vi "DAC_C2_Continu.vi"() -> ()   [LabVIEW 2015]
uses:
  <vilib>/DAQmx/read.llb/DAQmx Read (Analog DBL 1Chan 1Samp).vi
  <vilib>/DAQmx/create/channels.llb/DAQmx Create Channel (AI-Voltage-Basic).vi
  <vilib>/DAQmx/configure/timing.llb/DAQmx Timing (Sample Clock).vi
  <vilib>/DAQmx/miscellaneous.llb/DAQmx Fill In Error Info.vi
panel:
  in  "stop":bool
  out "data":dbl(graph)
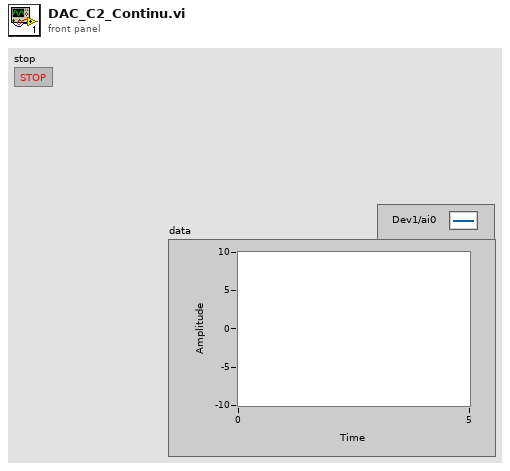
[diagram p1: front panel]
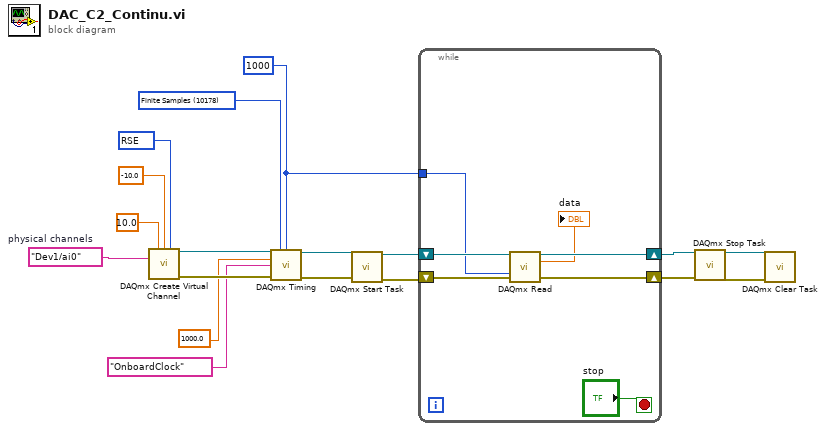
[diagram p0: block diagram]
diagram:
  w5 = 1000 ("samples per channel")
  w14 = 10178 items=["Finite Samples"=10178, "Continuous Samples"=10123, "Hardware Timed Single Point"=12522] ("sample mode")
  w15 = tag "Dev1/ai0"  # physical channels
  w18 = 10083 items=["Default"=-1, "RSE"=10083, "NRSE"=10078, "Differential"=10106, "Pseudodifferential"=12529] ("input terminal configuration")
  n1 = call-poly <vilib>:"DAQmx Create Virtual Channel.vi"("maximum value"=10.0, "minimum value"=-10.0, "input terminal configuration"=w18, "physical channels"=w15) -> ("task out"=w13:refnum<k21>, "error out"=w12:errorcluster)  [unwired: 10 in]
  n2 = call-poly <vilib>:"DAQmx Timing.vi"("task/channels in"=w13, "sample mode"=w14, "samples per channel"=w5, "rate"=1000.0, "source"=tag "OnboardClock", "error in"=w12) -> ("task out"=w9:refnum<k21>, "error out"=w7:errorcluster)  [unwired: 8 in]
  n3 = call <vilib>:"DAQmx Start Task.vi"("task/channels in"=w9, "error in"=w7) -> ("task out"=w8:refnum<k21>, "error out"=w6:errorcluster)  [unwired: 12 in]
  n4 = while {
    tunnel: w5 -> [w23]
    shift-right: [w21] -> w3
    shift-left: w8 -> [w25]
    shift-right: [w22] -> w4
    shift-left: w6 -> [w24]
    stop <- "stop" stop-if-true
    n5 = call-poly <vilib>:"DAQmx Read.vi"("task/channels in"=w25, "timeout"=w23, "error in"=w24) -> ("task out"=w21:refnum<k21>, "data"=→"data":dbl, "error out"=w22:errorcluster)  [unwired: 10 in]
  }
  n6 = call <vilib>:"DAQmx Stop Task.vi"("task/channels in"=w3, "error in"=w4) -> ("task out"=w2:refnum<k21>, "error out"=w1:errorcluster)  [unwired: 12 in]
  n7 = call <vilib>:"DAQmx Clear Task.vi"("task in"=w2, "error in"=w1) -> ()  [unwired: 13 in, 1 out]
